vi "Send Host Stream Command Stop.vi"(8 "error in (no error)":errorcluster, 11 "Cmd Q":refnum<queue>) -> (0 "error out":errorcluster)   [LabVIEW 2019, in "CAN Stream Support Workspace Shared.lvlib"]
uses:
  CAN Stream Support Workspace Shared.lvlib
  Types/Host Stream Queue Type.ctl
  Types/Host Stream Queue Command.ctl
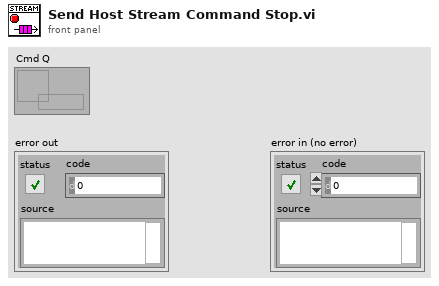
[diagram p1: front panel]
types:
  T1 = typedef "CAN Stream Support Workspace Shared.lvlib/Host Stream Queue Type.ctl" = cluster{"Cmd":T2, "Target IP Address":string, "Addon":string}
  T2 = typedef "CAN Stream Support Workspace Shared.lvlib/Host Stream Queue Command.ctl" = enum8{"Start Stream", "Stop Stream", "Exit"}
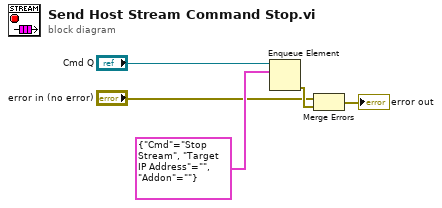
[diagram p0: block diagram]
diagram:
  n1 = Enqueue Element(queue="Cmd Q", element=T1 {"Cmd"=enum."Stop Stream", "Target IP Address"="", "Addon"=""}) -> (error out=w3:errorcluster)  [unwired: 2 in, 2 out]
  n2 = Merge Errors("error in (no error)", w3) -> (→"error out":errorcluster)
